vi "MeasureRMS.vi"() -> ()   [LabVIEW 2014]
uses:
  <vilib>/measure/madcrms.llb/Basic Averaged DC-RMS for N Chan.vi
  <vilib>/measure/NI_MAPro.lvlib
panel:
  out "RMS":dbl[](array[numeric]) format="%.2p"
  in  "stop":bool
  out "Waveform Graph":dynamicdata(graph)
  in  "Digitizing Parameters":T1
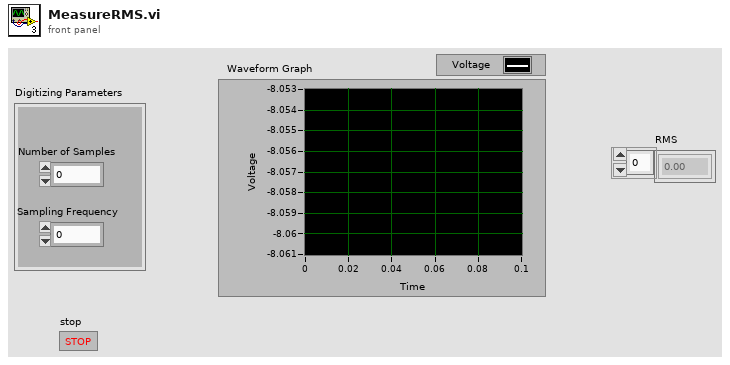
[diagram p1: front panel]
types:
  T1 = cluster{"Number of Samples":dbl, "Sampling Frequency":dbl}
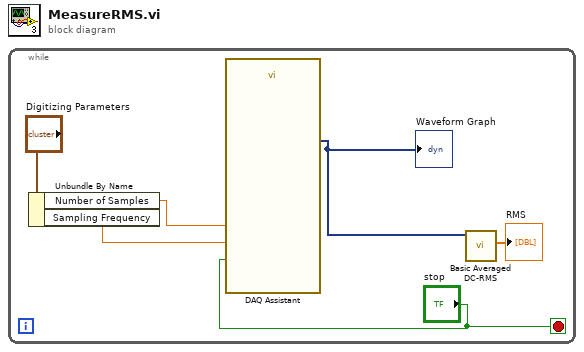
[diagram p0: block diagram]
diagram:
  n1 = while {
    stop <- "stop" stop-if-true
    n2 = Unbundle By Name("Digitizing Parameters") -> ("Number of Samples"=w5:dbl, "Sampling Frequency"=w4:dbl)
    n3 = call "DAQ Assistant"("rate"=w4, "number of samples"=w5, "stop (T)"="stop") -> ("data"=w1:dynamicdata)  [unwired: 14 in, 2 out]
    "Waveform Graph" <- w1
    n4 = call-poly <vilib>:"Basic Averaged DC-RMS.vi"("signals in"=w1) -> ("RMS values"=→"RMS":dbl[])  [unwired: 7 in, 3 out]
  }
